vi "extract Tilt value(SubVI).vi"(6 "0.1/0.01":bool, 8 "error in (no error)":errorcluster, 9 "Time out?":bool, 11 "Pelco-D response":string) -> (0 "error out":errorcluster, 3 "tilt1":dbl)   [LabVIEW 2018]
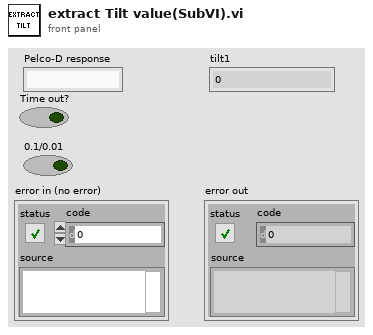
[diagram p1: front panel]
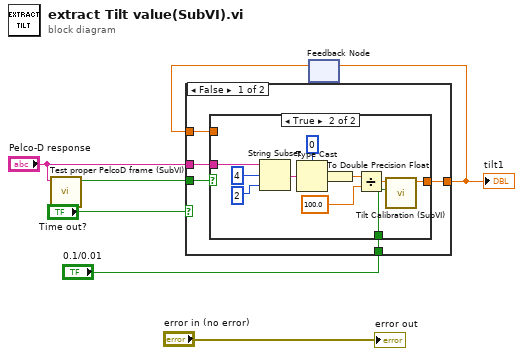
[diagram p0: block diagram]
diagram:
  n1 = call "Test proper PelcoD frame (SubVI).vi"("Pelco-D frame"="Pelco-D response") -> ("Proper?"=w2:bool)  [unwired: 10 in]
  n2 = feedback #1() -> (w5:dbl)  [unwired: 1 in]
  n3 = case shown="False" "Time out?" {
    tunnel: [w12 w25] -> w6
    tunnel: w5 -> [w11 w25]
    tunnel: "0.1/0.01" -> [w10 _]
    tunnel: w2 -> [w9 _]
    tunnel: "Pelco-D response" -> [w8 _]
    frame False {
      n4 = case shown="True" w9 {
        tunnel: w8 -> [_ w18]
        tunnel: [w13 w17] -> w12
        tunnel: w11 -> [w13 _]
        tunnel: w10 -> [_ w14]
        frame False {
        }
        frame True {
          n5 = String Subset(string=w18, offset (0)=4, length (rest)=2 ("length (rest)")) -> (substring=w19:string)
          n6 = Type Cast(type=u16 0, x=w19) -> (*(type *) &x=w16:u16)
          n7 = To Double Precision Float(number=w16) -> (double precision float=w15:dbl)
          n8 = Divide(x=w15, y=100.0) -> (x/y=w24:dbl)
          n9 = call "Tilt Calibration (SubVI).vi"("0.1/0.01"=w14, "tilt(360)"=w24) -> ("tilt"=w17:dbl)  [unwired: 9 in]
        }
      }
    }
    frame True {
      # "Time Out: SKIPPED"
    }
  }
  "tilt1" <- w6
  n10 = feedback-in #1(w6) -> ()
  "error out" <- "error in (no error)"
